vi "receive loop callback.vi"(4 "queue":refnum<queue>, 5 "Event Data":cluster{"msg in":string}, 6 "User Event Ref":refnum<user-event>, 7 "Event Common Data":T2 {"Event Source" items=["LabVIEW UI"=0, "ActiveX"=1, "User Event"=25]}) -> ()   [LabVIEW 2013, in "lvnano.lvlib"]
uses:
  <vilib>/event_ctls.llb/eventsource.ctl
  lvnano.lvlib
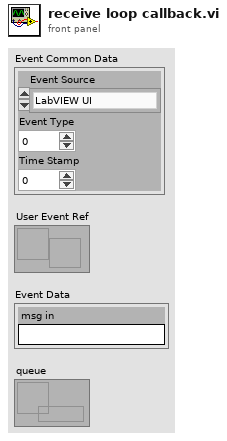
[diagram p1: front panel]
types:
  T1 = typedef "eventsource.ctl" = u32
  T2 = cluster{"Event Source":T1, "Event Type":u32, "Time Stamp":u32}
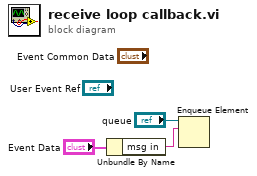
[diagram p0: block diagram]
diagram:
  n1 = Unbundle By Name("Event Data") -> ("msg in"=w2:string)
  n2 = Enqueue Element(queue="queue", element=w2) -> ()  [unwired: 2 in, 3 out]
